vi "AuxLockFluo.vi"(4 "XAOMsetting 2":refnum<vi>, 6 "Camera?":bool, 7 "FluoRefIn":refnum<vi>, 8 "error in":errorcluster, 9 "Completed loops in":u32, 11 "fluo in":dbl) -> (0 "error out":errorcluster, 1 "Completed loops out":u32, 2 "fluo normalized":dbl, 3 "fl lock bools":T2)   [LabVIEW 2019]
uses:
  controls/FluoSettings.ctl
  controls/xAOMSettings/XAOMsetting.xctl
  <vilib>/Utility/error.llb/Error Cluster From Error Code.vi
  <vilib>/rvi/errors/niLvFpgaAdjustHostInterfaceError.vi
  <vilib>/rvi/interface/nirviReadWriteControl/nirviReadWriteControl.xnode
  NiFpgaLv.dll
  <vilib>/rvi/interface/Simulation/niFpgaSimulationCallBeginRW.vi
panel:
  in  "XAOMsetting":T1(xcontrol)
  in  "FluoCtrl":T3
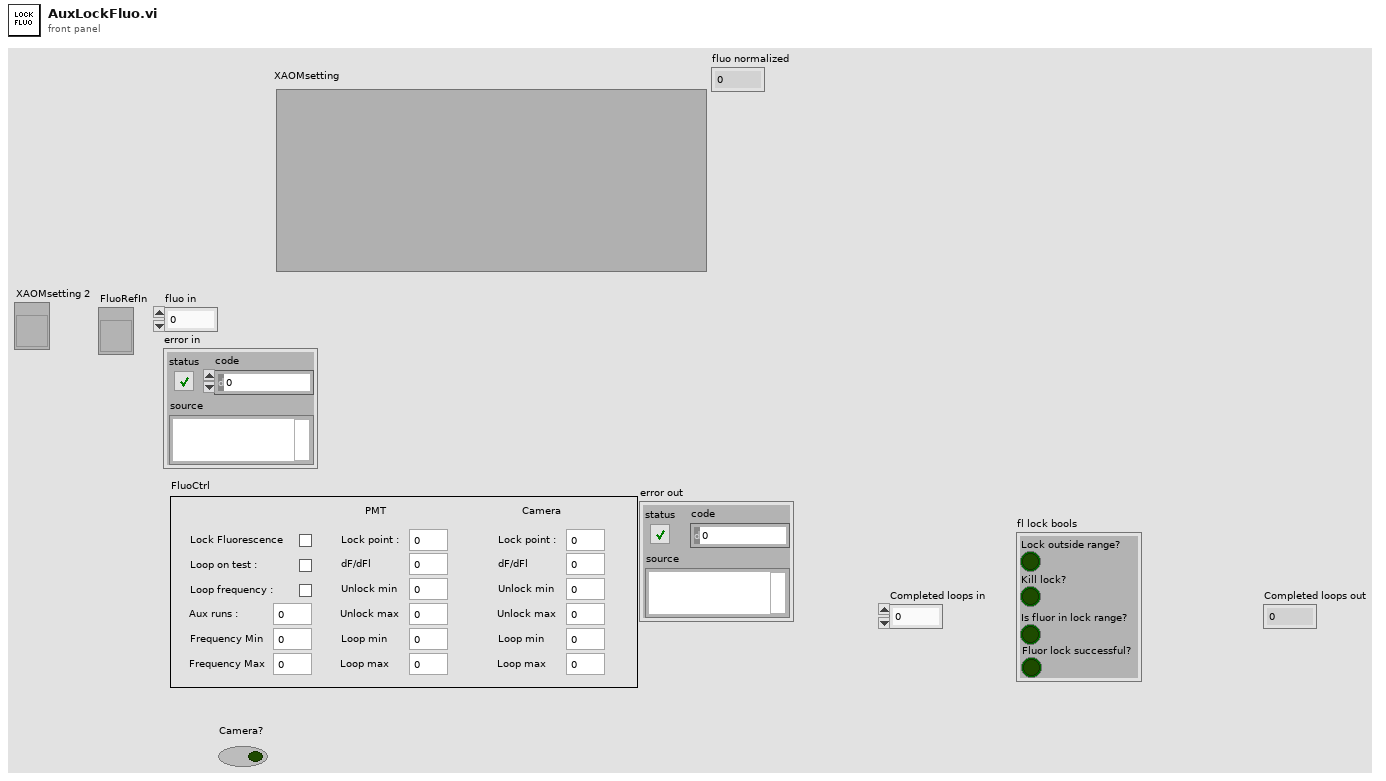
[diagram p1: front panel]
types:
  T1 = cluster{"HighPowerNum":dbl, "LowPowerNum":dbl, "PIDnum":dbl, "DeltaFreq":dbl, "BaseFreq":dbl, "AOMout":dbl, "ButtonSelected":enum16{"PID", "Low", "High"}, "AO3":bool}
  T2 = cluster{"Lock outside range?":bool, "Kill lock?":bool, "Is fluor in lock range?":bool, "Fluor lock successful?":bool}
  T3 = typedef "FluoSettings.ctl" = cluster{"Lock Fluorescence":bool, "Aux runs : ":i32, "Loop on test :":bool, "Loop frequency : ":bool, "Frequency Min":dbl, "Frequency Max":dbl, "PMT":cluster{"Lock point : ":dbl, "dF/dFl":dbl, "Unlock min":dbl, "Unlock max":dbl, "Loop min":dbl, "Loop max":dbl}, "Camera":cluster{"Lock point : ":dbl, "dF/dFl":dbl, "Unlock min":dbl, "Unlock max":dbl, "Loop min":dbl, "Loop max":dbl}}
  T4 = cluster{"Lock point : ":dbl, "dF/dFl":dbl, "Unlock min":dbl, "Unlock max":dbl, "Loop min":dbl, "Loop max":dbl}
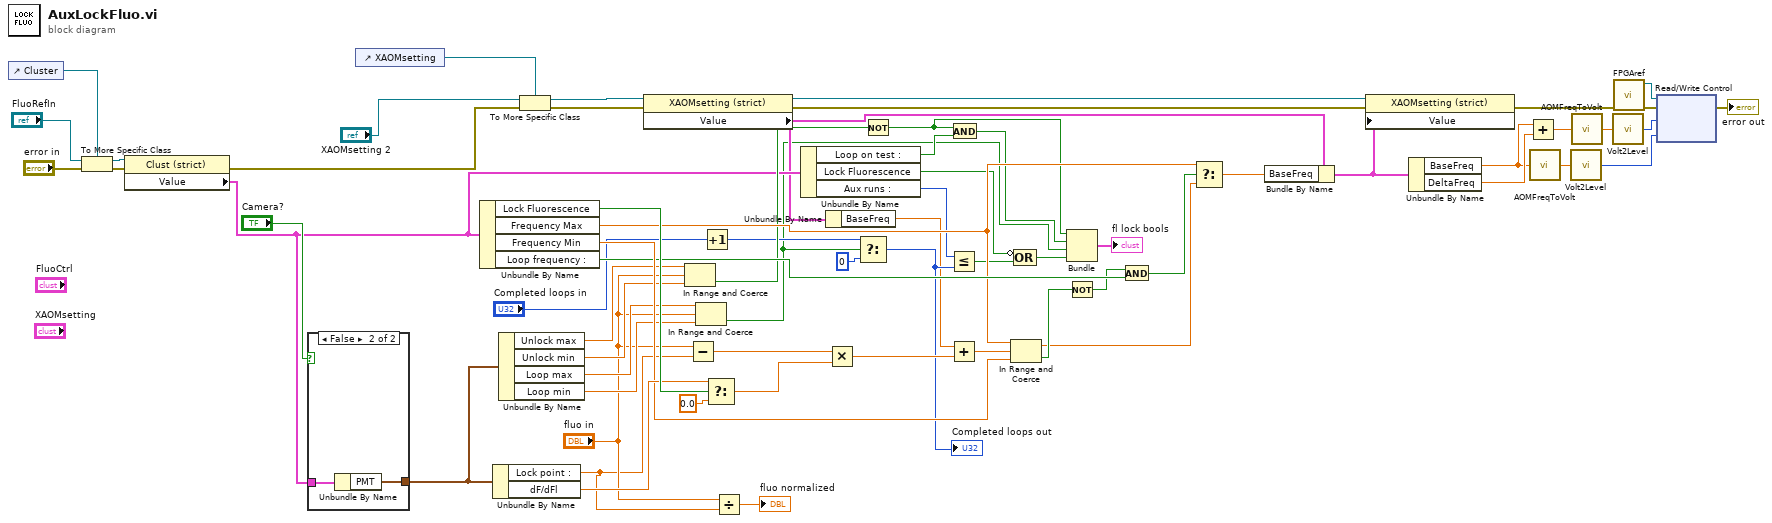
[diagram p0: block diagram]
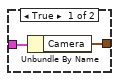
[diagram p2: hidden frame]
diagram:
  n1 = control-ref of="Cluster"() -> (w64:refnum<vi>)
  n2 = To More Specific Class(target class=w64, reference="FluoRefIn", error in="error in") -> (specific class reference=w63:refnum<vi>, error out=w7:errorcluster)
  n3 = property class="Clust (strict)"(reference=w63, error in=w7) -> (error out=w8:errorcluster, "Value"=w33:T3)  [unwired: 1 out]
  n4 = case shown="False" "Camera?" {
    tunnel: w33 -> [w67 w69]
    tunnel: [w66 w68] -> w47
    frame True {
      n5 = Unbundle By Name(w67) -> ("Camera"=w66:T4)
    }
    frame False {
      n6 = Unbundle By Name(w69) -> ("PMT"=w68:T4)
    }
  }
  n7 = control-ref of="XAOMsetting"() -> (w4:refnum<vi>)
  n8 = Unbundle By Name(w33) -> ("Lock Fluorescence"=w61:bool, "Frequency Max"=w48:dbl, "Frequency Min"=w56:dbl, "Loop frequency :"=w52:bool)
  n9 = Unbundle By Name(w47) -> ("Lock point :"=w2:dbl, "dF/dFl"=w60:dbl)
  n10 = Unbundle By Name(w47) -> ("Unlock max"=w46:dbl, "Unlock min"=w45:dbl, "Loop max"=w44:dbl, "Loop min"=w43:dbl)
  n11 = To More Specific Class(target class=w4, reference="XAOMsetting 2", error in=w8) -> (specific class reference=w23:refnum<vi>, error out=w9:errorcluster)
  n12 = property class="XAOMsetting (strict)"(reference=w23, error in=w9) -> (reference out=w18:refnum<vi>, error out=w19:errorcluster, "Value"=w21:T1)
  n13 = In Range and Coerce(upper limit=w46, x="fluo in", lower limit=w45) -> (In Range?=w42:bool)  [unwired: 1 out]
  n14 = Subtract(x="fluo in", y=w2) -> (x-y=w57:dbl)
  n15 = In Range and Coerce(upper limit=w44, x="fluo in", lower limit=w43) -> (In Range?=w13:bool)  [unwired: 1 out]
  n16 = Increment(x="Completed loops in") -> (x+1=w36:u32)
  n17 = Select(t=w60, s=w61, f=0.0) -> (s? t:f=w58:dbl)
  n18 = Divide(x="fluo in", y=w2) -> (x/y=→"fluo normalized":dbl)
  n19 = Unbundle By Name(w33) -> ("Loop on test :"=w32:bool, "Lock Fluorescence"=w30:bool, "Aux runs :"=w31:i32)
  n20 = Unbundle By Name(w21) -> ("BaseFreq"=w22:dbl)
  n21 = Multiply(x=w57, y=w58) -> (x*y=w54:dbl)
  n22 = Select(t=w36, s=w13, f=u32 0) -> (s? t:f=w34:u32)
  "Completed loops out" <- w34
  n23 = Not(x=w42) -> (.not. x?=w40:bool)
  n24 = Less Or Equal?(x=w31, y=w34) -> (x <= y?=w37:bool)
  n25 = Add(x=w22, y=w54) -> (x+y=w55:dbl)
  n26 = And(x=w40, y=w32) -> (x .and. y?=w39:bool)
  n27 = In Range and Coerce(upper limit=w48, x=w55, lower limit=w56) -> (coerced(x)=w49:dbl, In Range?=w53:bool)
  n28 = Compound Arithmetic op=OR(invert w30, w37) -> (w29:bool)
  n29 = Bundle(w40, w39, w13, w29) -> (→"fl lock bools":cluster{bool, bool, bool, bool})  [unwired: 1 in]
  n30 = Not(x=w53) -> (.not. x?=w51:bool)
  n31 = And(x=w51, y=w52) -> (x .and. y?=w50:bool)
  n32 = Select(t=w48, s=w50, f=w49) -> (s? t:f=w20:dbl)
  n33 = Bundle By Name(cluster=w21, "BaseFreq"=w20) -> (w17:T1)
  n34 = property class="XAOMsetting (strict)"(reference=w18, error in=w19, "Value"=w17) -> (error out=w12:errorcluster)  [unwired: 1 out]
  n35 = Unbundle By Name(w17) -> ("BaseFreq"=w14:dbl, "DeltaFreq"=w16:dbl)
  n36 = Add(x=w14, y=w16) -> (x+y=w15:dbl)
  n37 = call "AOMFreqToVolt.vi"("AOM freq"=w14) -> ("AOM voltage"=w25:dbl)
  n38 = call "Volt2Level.vi"("voltage /V"=w25) -> ("level"=w24:i16)
  n39 = call "AOMFreqToVolt.vi"("AOM freq"=w15) -> ("AOM voltage"=w27:dbl)
  n40 = call "Volt2Level.vi"("voltage /V"=w27) -> ("level"=w26:i16)
  n41 = call "FPGAref.vi"("error in"=w12) -> ("error out"=w11:errorcluster, "FPGA VI Reference Out 2"=w28:refnum<k20>)  [unwired: 5 in]
  n42 = xnode "Read/Write Control"("FPGA VI Reference In"=w28, "error in"=w11, "AO3 on"=w26, "AO3 off"=w24) -> ("error out"=→"error out":errorcluster)  [unwired: 1 out]
